vi "Actor Core.vi"(8 "error in":errorcluster, 11 "Nested in":refnum<class "Coca.lvclass">) -> (0 "error out":errorcluster, 3 "Actor out":refnum<class "Actor.lvclass">)   [LabVIEW 2020, in "Coca.lvlib" / "Coca.lvclass"]
doc: "(<B>Filename</B>: Actor Framework.lvlib:Actor.lvclass:Actor Core.vi)\n\nReceives messages to the actor, reacts to them, and initiates any error handling that may shut the actor down.\n\nDescendant classes may override this VI to append parallel tasks for the actor to complete while it handles messages. Overrides use the Call Parent Method node."
uses:
  Coca.lvclass
  C:/Program Files (x86)/National Instruments/LabVIEW 2020/vi.lib/ActorFramework/Actor/Actor.lvclass
  <vilib>/ActorFramework/Actor/Actor.lvclass
  <vilib>/ActorFramework/Actor/Actor.lvclass/Actor.ctl
  <vilib>/ActorFramework/Message Enqueuer/Message Enqueuer.lvclass/Message Enqueuer.ctl
  Coca.lvclass/Coca.ctl
  Coca Messages/Send Product Msg/Send Product Msg.lvclass/Send Product Msg.ctl
  <vilib>/ActorFramework/Message Enqueuer/Init from Existing Queue.vi
  <vilib>/ActorFramework/Message Enqueuer/Enqueue.vi
  <vilib>/ActorFramework/Stop Msg/Stop Msg.lvclass
  C:/Program Files (x86)/National Instruments/LabVIEW 2020/vi.lib/ActorFramework/Message/Message.lvclass
  Coca Messages/Send Product Msg/Send Product Msg.lvclass
  <vilib>/ActorFramework/Message Priority Queue/Priority Enqueue.vi
  <vilib>/ActorFramework/Message Enqueuer/Message Enqueuer.lvclass
  Coca Messages/Comprar Msg/Comprar Msg.lvclass
panel:
  in  "Productos":i32(listbox)
  in  "Comprar":bool
  # "Coca"
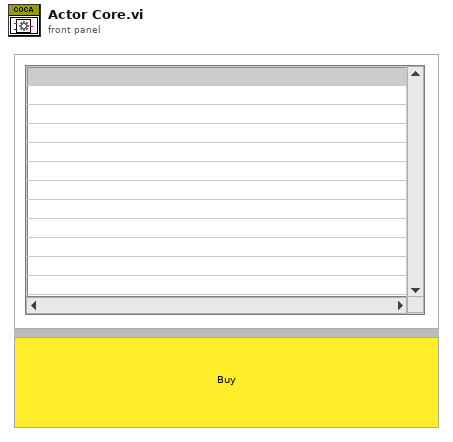
[diagram p1: front panel]
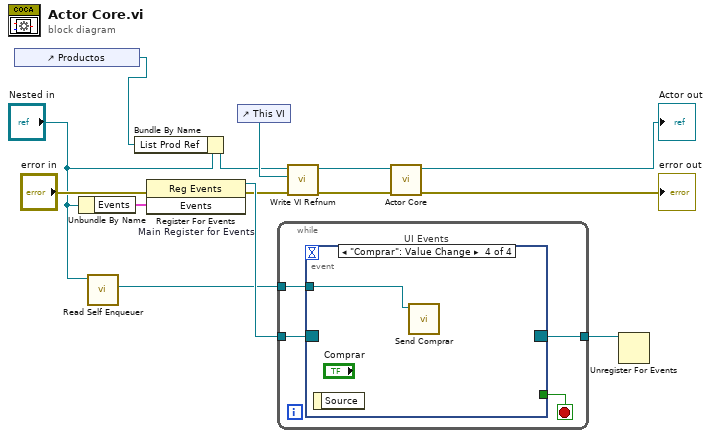
[diagram p0: block diagram]
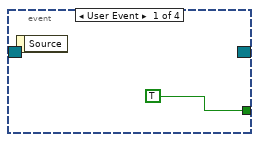
[diagram p2: hidden frame]
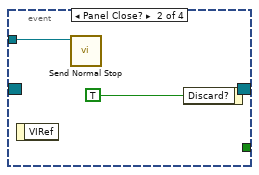
[diagram p3: hidden frame]
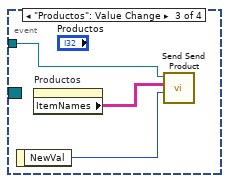
[diagram p4: hidden frame]
diagram:
  n1 = control-ref of="Productos"() -> (w1:refnum<vi>)
  n2 = Unbundle By Name("Nested in") -> ("Events"=w11:cluster{"Stop":refnum<user-event>})
  n3 = call <vilib>:"Read Self Enqueuer.vi"("Actor"="Nested in") -> ("Self Enqueuer"=w9:refnum<class "Message Enqueuer.lvclass">)  [unwired: 10 in]
  n4 = Bundle By Name(cluster="Nested in", "List Prod Ref"=w1) -> (w2:refnum<class "Coca.lvclass">)
  n5 = register-events "Main Register for Events"(error in="error in", w11) -> (reference out=w12:refnum<event-registration>, error out=w6:errorcluster)  [unwired: 1 in]
  n6 = control-ref of="This VI"() -> (w3:refnum<vi>)
  n7 = while {
    tunnel: w12 -> [w18]
    tunnel: [w16] -> w10
    tunnel: w9 -> [w15]
    stop <- w17 stop-if-true
    n8 = event "UI Events" shown="[3] \"Comprar\": Value Change" {
      selector: w18 -> [_ _ _ _]
      dyn-events: [_ _ _ _] -> w16
      timeout: _ -> [_ _ _ _]
      tunnel: [TRUE _ _ _] -> w17
      tunnel: w15 -> [_ w20 w24 w25]
      event User Event {
        n9 = event-data() -> ()  [unwired: 1 in, 1 out]
      }
      event Panel Close? {
        n10 = event-data() -> ()  [unwired: 1 in, 1 out]
        n11 = call <vilib>:"Send Normal Stop.vi"("Message Enqueuer"=w20) -> ()  [unwired: 10 in, 1 out]
        n12 = event-data("Discard?"=TRUE) -> ()  [unwired: 1 in, 1 out]
      }
      event "Productos": Value Change {
        n13 = event-data() -> ("NewVal"=w22:i32)  [unwired: 1 in]
        n14 = property on="Productos" class="MCListbox (strict)"() -> ("ItemNames"=w23:string[][])  [unwired: 2 in, 2 out]
        n15 = call "Send Send Product.vi"("index"=w22, "Item Names"=w23, "Message Enqueuer"=w24) -> ()  [unwired: 7 in, 2 out]
      }
      event "Comprar": Value Change {
        n16 = event-data() -> ()  [unwired: 1 in, 1 out]
        n17 = call "Send Comprar.vi"("Message Enqueuer"=w25) -> ()  [unwired: 9 in, 2 out]
      }
    }
  }
  n18 = call "Write VI Refnum.vi"("error in (no error)"=w6, "VI Refnum"=w3, "Coca in"=w2) -> ("error out"=w4:errorcluster, "Coca out"=w5:refnum<class "Coca.lvclass">)  [unwired: 7 in]
  n19 = call-parent "Actor Core.vi"("error in"=w4, "Actor in"=w5) -> ("error out"=→"error out":errorcluster, "Actor out"=→"Actor out":refnum<class "Actor.lvclass">)  [unwired: 8 in]
  n20 = Unregister For Events(event registration refnum=w10) -> ()  [unwired: 1 in, 1 out]
